vi "Write Coil Moxa.vi"(3 "error in":errorcluster, 4 "coil to write":bool, 5 "Coil":u16) -> (0 "error IO":errorcluster, 1 "State":bool)   [LabVIEW 2022 SP3]
uses:
  <vilib>/NI/Modbus Library/API/Master/Modbus Master.lvclass
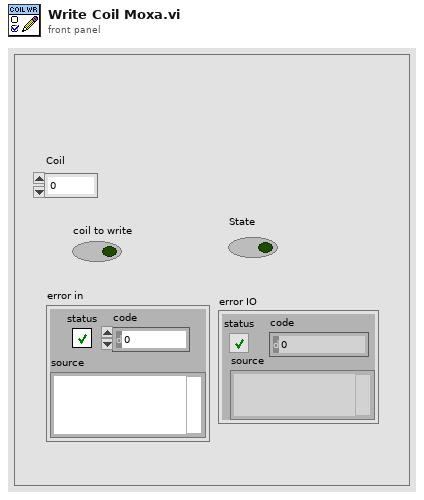
[diagram p1: front panel]
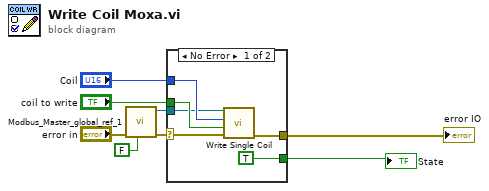
[diagram p0: block diagram]
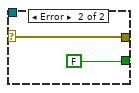
[diagram p2: hidden frame]
diagram:
  n1 = call "Modbus_Master_global_ref_1.vi"("Read:F/Wirte:T"=FALSE, "error in (no error) 2"="error in") -> ("error out 2"=w2:errorcluster, "Modbus Master out"=w1:refnum<class "Modbus Master.lvclass">)  [unwired: 8 in]
  n2 = case shown="No Error" w2 {
    selector: w2 -> [w9 w15]
    tunnel: "Coil" -> [w11 _]
    tunnel: "coil to write" -> [w12 _]
    tunnel: [w14 w15] -> w6
    tunnel: [TRUE FALSE] -> w5
    tunnel: w1 -> [w10 _]
    frame No Error {
      n3 = call-dynamic "Write Single Coil.vi"("error in"=w9, "coil to write"=w12, "address"=w11, "Modbus master in"=w10) -> ("error out"=w14:errorcluster)  [unwired: 6 in, 1 out]
    }
    frame Error {
    }
  }
  "State" <- w5
  "error IO" <- w6
